vi "Losuj z zakresu.vi"(8 "error in (no error)":errorcluster, 11 "Zakr":dbl) -> (0 "error out":errorcluster, 3 "Wart":i16)   [LabVIEW 2014, in "Swiat.lvclass"]
uses:
  Swiat.lvclass
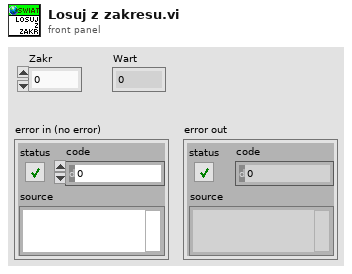
[diagram p1: front panel]
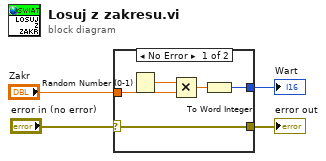
[diagram p0: block diagram]
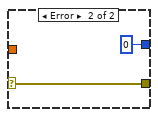
[diagram p2: hidden frame]
diagram:
  n1 = case shown="No Error" "error in (no error)" {
    selector: "error in (no error)" -> [w5 w11]
    tunnel: [w9 i16 0] -> w4
    tunnel: "Zakr" -> [w7 _]
    tunnel: [w5 w11] -> w1
    frame No Error {
      n2 = Random Number (0-1)() -> (number: 0 to 1=w8:dbl)
      n3 = Multiply(x=w8, y=w7) -> (x*y=w6:dbl)
      n4 = To Word Integer(number=w6) -> (16bit integer=w9:i16)
    }
    frame Error {
    }
  }
  "Wart" <- w4
  "error out" <- w1
